vi "Get User Input.vi"(7 "Dialog Message":string) -> (4 "User Input":string, 15 "Canceled?":bool)   [LabVIEW 2016]
uses:
  <vilib>/Utility/miscctls.llb/LVPointTypeDef.ctl
panel:
  in  "Get User Input":string caption="This is a Test"
  in  "Cancel":bool
  in  "Done":bool
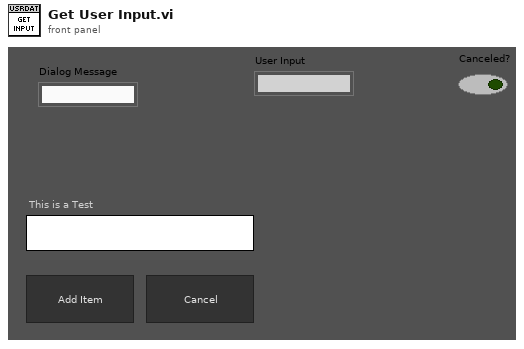
[diagram p1: front panel]
types:
  T1 = enum16{"Always On", "Always Off", "Off While Running"}
  T2 = typedef "LVPointTypeDef.ctl" = cluster{"Horizontal":i16, "Vertical":i16}
  T3 = typedef "LVRectTypeDef.ctl" = cluster{"Left":i16, "Top":i16, "Right":i16, "Bottom":i16}
  T4 = typedef "LVBoundsTypeDef.ctl" = cluster{"Width":u32, "Height":u32}
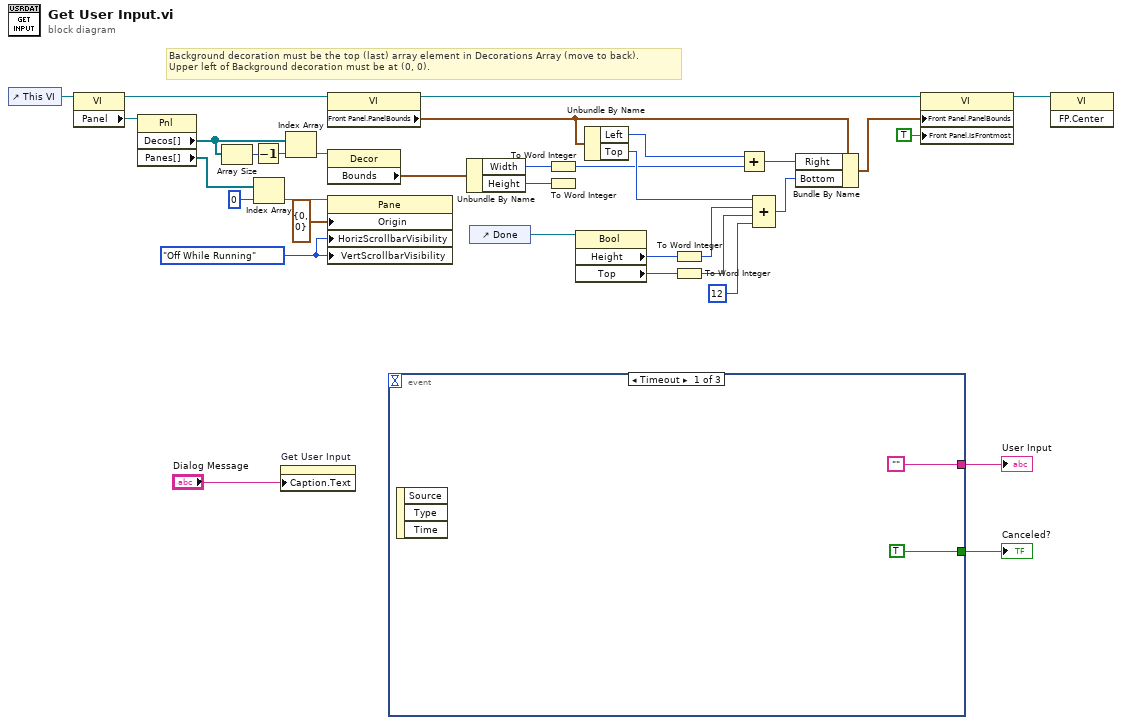
[diagram p0: block diagram]
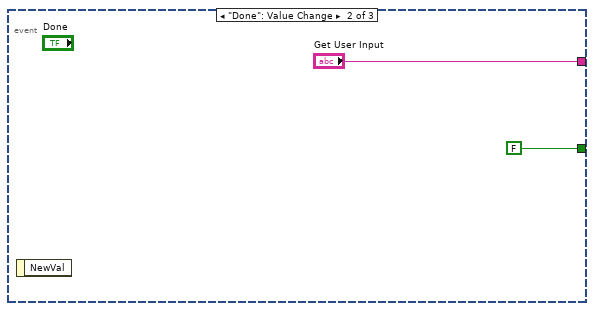
[diagram p2: hidden frame]
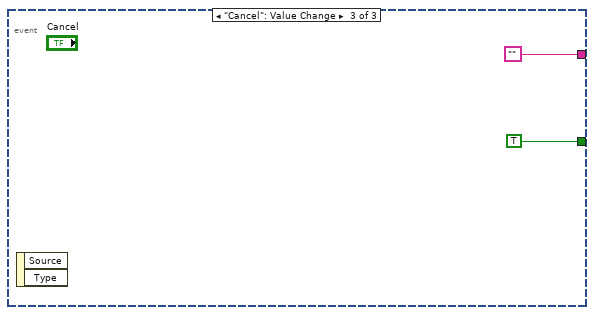
[diagram p3: hidden frame]
diagram:
  w17 = T1."Off While Running" ("Vertical Scrollbar Visibility")
  # "Background decoration must be the top (last) array element in Decorations Array (move to back).\nUpper left of Background decoration must be at (0, 0)."
  n1 = control-ref of="This VI"() -> (w9:refnum<vi>)
  n2 = property class="VI"(reference=w9) -> (reference out=w18:refnum<vi>, "Panel"=w10:refnum<vi>)  [unwired: 1 in, 1 out]
  n3 = property class="Pnl"(reference=w10) -> ("Decos[]"=w8:refnum<vi>[], "Panes[]"=w14:refnum<vi>[])  [unwired: 1 in, 2 out]
  n4 = Array Size(array=w8) -> (size(s)=w6:i32)
  n5 = Decrement(x=w6) -> (x-1=w7:i32)
  n6 = Index Array(array=w14, index=0) -> (element=w13:refnum<vi>)
  n7 = property on="Get User Input" class="Str"("Caption.Text"="Dialog Message") -> ()  [unwired: 2 in, 2 out]
  n8 = Index Array(array=w8, index=w7) -> (element=w16:refnum<vi>)
  n9 = property class="VI"(reference=w18) -> (reference out=w20:refnum<vi>, "Front Panel.PanelBounds"=w21:T3)  [unwired: 1 in, 1 out]
  n10 = property class="Decor"(reference=w16) -> ("Bounds"=w19:T4)  [unwired: 1 in, 2 out]
  n11 = property class="Pane"(reference=w13, "Origin"=T2 {"Horizontal"=0, "Vertical"=0}, "HorizScrollbarVisibility"=w17, "VertScrollbarVisibility"=w17) -> ()  [unwired: 1 in, 2 out]
  n12 = event shown="[0] Timeout" {
    selector: _ -> [_ _ _]
    dyn-events: _ -> [_ _ _]
    timeout: _ -> [_ _ _]
    tunnel: ["" "Get User Input" ""] -> w2
    tunnel: [TRUE FALSE TRUE] -> w1
    event Timeout {
      n13 = event-data() -> ()  [unwired: 1 in, 3 out]
    }
    event "Done": Value Change {
      n14 = event-data() -> ()  [unwired: 1 in, 1 out]
    }
    event "Cancel": Value Change {
      n15 = event-data() -> ()  [unwired: 1 in, 2 out]
    }
  }
  "Canceled?" <- w1
  "User Input" <- w2
  n16 = Unbundle By Name(w19) -> ("Width"=w24:u32, "Height"=w27:u32)
  n17 = control-ref of="Done"() -> (w11:refnum<vi>)
  n18 = To Word Integer(number=w24) -> (16bit integer=w26:i16)
  n19 = To Word Integer(number=w27) -> ()  [unwired: 1 out]
  n20 = property class="Bool"(reference=w11) -> ("Height"=w29:u32, "Top"=w30:i32)  [unwired: 1 in, 2 out]
  n21 = Unbundle By Name(w21) -> ("Left"=w23:i16, "Top"=w34:i16)
  n22 = To Word Integer(number=w29) -> (16bit integer=w32:i16)
  n23 = To Word Integer(number=w30) -> (16bit integer=w33:i16)
  n24 = Add(x=w23, y=w26) -> (x+y=w25:i16)
  n25 = Compound Arithmetic op=ADD(w34, w32, w33, i16 12 ("y")) -> (w28:i16)
  n26 = Bundle By Name(cluster=w21, "Right"=w25, "Bottom"=w28) -> (w22:T3)
  n27 = property class="VI"(reference=w20, "Front Panel.PanelBounds"=w22, "Front Panel.IsFrontmost"=TRUE ("Front Panel Window:Is Frontmost")) -> (reference out=w4:refnum<vi>)  [unwired: 1 in, 1 out]
  n28 = invoke class="VI" method="FP.Center"(reference=w4) -> ()  [unwired: 2 in, 3 out]
